vi "Create.vi"(8 "error in (no error)":errorcluster, 10 "Expected":i32) -> (0 "error out":errorcluster, 3 "Count":refnum<class "Count.lvclass">)   [LabVIEW 2017, in "Transparent Assertions.lvlib" / "Count.lvclass"]
uses:
  Count.lvclass
  Count.lvclass/Count.ctl
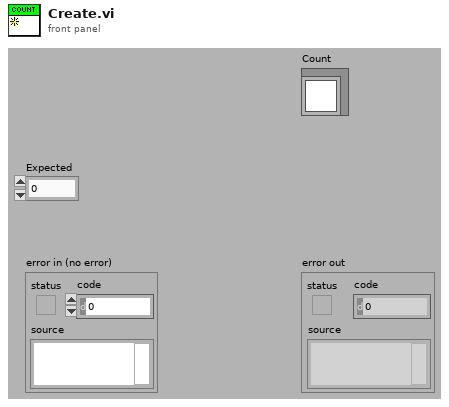
[diagram p1: front panel]
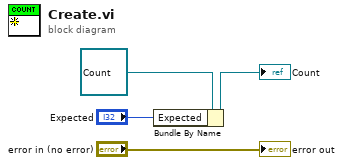
[diagram p0: block diagram]
diagram:
  n1 = Bundle By Name(cluster=refnum<class "Count.lvclass"> refnum ("Count In"), "Expected"="Expected") -> (→"Count":refnum<class "Count.lvclass">)
  "error out" <- "error in (no error)"
